vi "Stop Core.vi"(10 "final error code":i32, 11 "Syringe in":refnum<class "Syringe.lvclass">) -> (3 "Syringe out":refnum<class "Syringe.lvclass">)   [LabVIEW 2015, in "AMS UI.lvlib" / "Syringe.lvclass"]
doc: "(<B>Filename</B>: Actor Framework.lvlib:Actor.lvclass:Stop Core.vi)\n\nDefines what the actor does before it stops. Use the <B>final error code</B> input to determine whether the actor shut down in response to an error.\n\nBy default, this method does nothing. A descendant class may override it to define behavior, such as shutting down any processes the actor initiated in its override of the Actor Core method."
uses:
  Syringe.lvclass
  Syringe.lvclass/Syringe.ctl
  AMS Gas Actor/AMS Gas Actor.lvclass
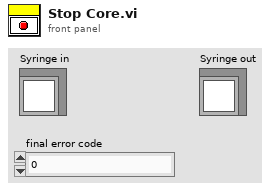
[diagram p1: front panel]
types:
  T1 = typedef "Sample Container.ctl" = cluster{"Sample In":refnum<k21>, "Sample Name":refnum<k21>, "Ti Cathode":refnum<k21>, "SampleQ":refnum<queue>}
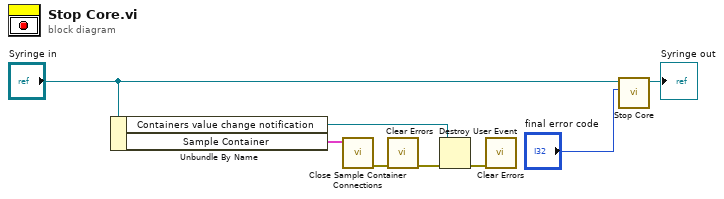
[diagram p0: block diagram]
diagram:
  n1 = Unbundle By Name("Syringe in") -> ("Containers value change notification"=w2:refnum<user-event>, "Sample Container"=w6:T1)
  n2 = call "Close Sample Container Connections.vi"("Container in"=w6) -> ("error out"=w5:errorcluster)  [unwired: 9 in, 1 out]
  n3 = call <vilib>:"Clear Errors.vi"("error in (no error)"=w5) -> ("error out"=w3:errorcluster)  [unwired: 5 in, 1 out]
  n4 = Destroy User Event(user event=w2, error in=w3) -> (error out=w1:errorcluster)
  n5 = call <vilib>:"Clear Errors.vi"("error in (no error)"=w1) -> ()  [unwired: 5 in, 2 out]
  n6 = call-parent "Stop Core.vi"("final error code"="final error code", "AMS Gas Actor in"="Syringe in") -> ("AMS Gas Actor out"=→"Syringe out":refnum<class "Syringe.lvclass">)  [unwired: 9 in]
